vi "Find Duplicate Test.vi"() -> (0 "error out":errorcluster, 2 "Success NO Duplicate":bool, 3 "Success Duplicate Detected":bool)   [LabVIEW 2014, in "SQLite tests.lvlib"]
doc: "Tests the Add Line and Remove Line functions."
uses:
  SQLite tests.lvlib
  <vilib>/NI/Tag Bus Module Framework/module configuration/TBM module configuration.lvclass
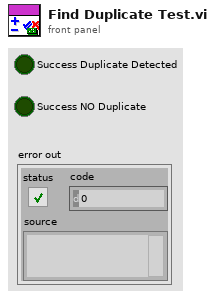
[diagram p1: front panel]
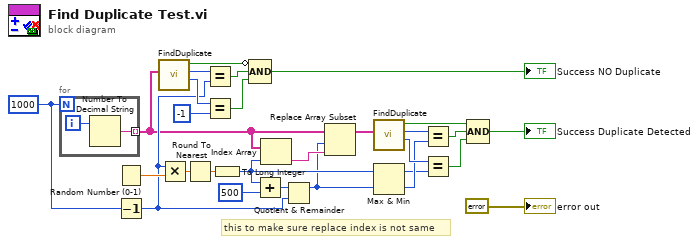
[diagram p0: block diagram]
diagram:
  w28 = 1000
  # "this to make sure replace index is not same"
  n1 = for {
    N: w28 -> [_]
    tunnel: [w29] -> w1 mode=indexing
    i -> [w30]
    n2 = Number To Decimal String(number=w30) -> (decimal integer string=w29:string)  [unwired: 1 in]
  }
  n3 = Random Number (0-1)() -> (number: 0 to 1=w27:dbl)
  n4 = Decrement(x=w28) -> (x-1=w6:i32)
  n5 = call <vilib>:"FindDuplicate.vi"("Array"=w1) -> ("Index 2"=w14:i32, "Index 1"=w16:i32, "Duplicate"=w10:bool)  [unwired: 8 in]
  n6 = Multiply(x=w6, y=w27) -> (x*y=w26:dbl)
  n7 = Round To Nearest(number=w26) -> (nearest integer value=w25:dbl)
  n8 = Equal?(x=w16, y=w6) -> (x = y?=w12:bool)
  n9 = Equal?(x=w14, y=-1 ("x")) -> (x = y?=w13:bool)
  n10 = To Long Integer(number=w25) -> (32bit integer=w5:i32)
  n11 = Compound Arithmetic op=AND(invert w10, w12, w13) -> (→"Success NO Duplicate":bool)
  n12 = Add(x=w5, y=500) -> (x+y=w7:i32)
  n13 = Index Array(array=w1, index=w5) -> (element=w24:string)
  n14 = Quotient & Remainder(x=w7, y=w6) -> (x-y*floor(x/y)=w4:i32)  [unwired: 1 out]
  n15 = Replace Array Subset(array=w1, new element=w24, index=w4) -> (w23:string[])
  n16 = call <vilib>:"FindDuplicate.vi"("Array"=w23) -> ("Index 2"=w19:i32, "Index 1"=w21:i32, "Duplicate"=w22:bool)  [unwired: 8 in]
  n17 = Max & Min(x=w5, y=w4) -> (max(x,y)=w2:i32, min(x,y)=w3:i32)
  n18 = Equal?(x=w21, y=w3) -> (x = y?=w20:bool)
  n19 = Equal?(x=w19, y=w2) -> (x = y?=w18:bool)
  n20 = Compound Arithmetic op=AND(w22, w20, w18) -> (→"Success Duplicate Detected":bool)
  "error out" <- errorcluster {"status"=FALSE, "code"=0, "source"=""} ("error out")
